vi "CMN_Numb2Hex.vi"(10 "input str":string) -> (0 "error":errorcluster, 1 "output hexa":string, 2 "remaining string":string)   [LabVIEW 2016]
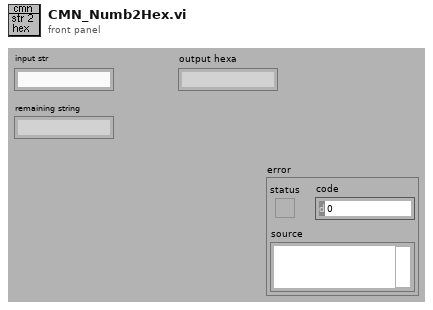
[diagram p1: front panel]
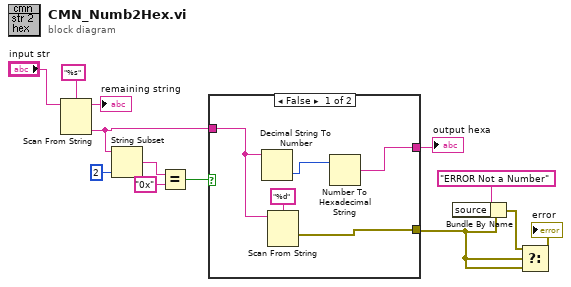
[diagram p0: block diagram]
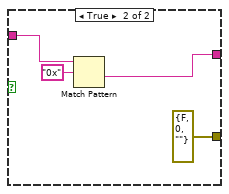
[diagram p2: hidden frame]
diagram:
  n1 = Scan From String(format string="%s", input string="input str") -> (remaining string=→"remaining string":string, output 1=w7:string)  [unwired: 2 in, 3 out]
  n2 = String Subset(string=w7, length (rest)=2 ("length (rest)")) -> (substring=w10:string)  [unwired: 1 out]
  n3 = Equal?(x=w10, y="0x") -> (x = y?=w8:bool)
  n4 = case shown="False" w8 {
    tunnel: w7 -> [w16 w22]
    tunnel: [w17 w20] -> w6
    tunnel: [w14 errorcluster {"status"=FALSE, "code"=0, "source"=""} ("error IO")] -> w2
    frame False {
      n5 = Decimal String To Number(string=w16) -> (number=w18:i32)  [unwired: 3 out]
      n6 = Scan From String(format string="%d", input string=w16) -> (error out=w14:errorcluster)  [unwired: 2 in, 4 out]
      n7 = Number To Hexadecimal String(2:w18) -> (0:w17:string)  [unwired: 1 out]
    }
    frame True {
      n8 = Match Pattern(string=w22, regular expression="0x") -> (after substring=w20:string)  [unwired: 4 out]
    }
  }
  "output hexa" <- w6
  n9 = Bundle By Name(cluster=w2, "source"="ERROR Not a Number") -> (w3:errorcluster)
  n10 = Select(t=w3, s=w2, f=w2) -> (s? t:f=→"error":errorcluster)
